vi "11.vi"() -> ()   [LabVIEW 2023]
uses:
  <vilib>/Utility/file.llb/Read Delimited Spreadsheet (string).vi
  <vilib>/Utility/file.llb/Write Delimited Spreadsheet (string).vi
panel:
  in  "stop":bool
  out "subarray 2":dbl[](array[numeric])
  out "x citit":dbl[](array[numeric])
  out "deleted portion":string[](array[string])
  out "array w/ subset deleted":string[][](array[string])
  out "XY Graph 2":cluster{dbl[], dbl[]}(graph)
  in  "desen":bool
  out "Y":dbl
  out "X":dbl
  out "subarray":string[](array[string])
  out "all rows":string[][](array[string])
  in  "citeste":bool
  in  "save":bool
  in  "b":dbl(slide) scale=0.0..10.0
  in  "a":dbl(slide) scale=0.0..10.0
  out "XY Graph":cluster{"X":dbl, "Y":dbl}[](graph)
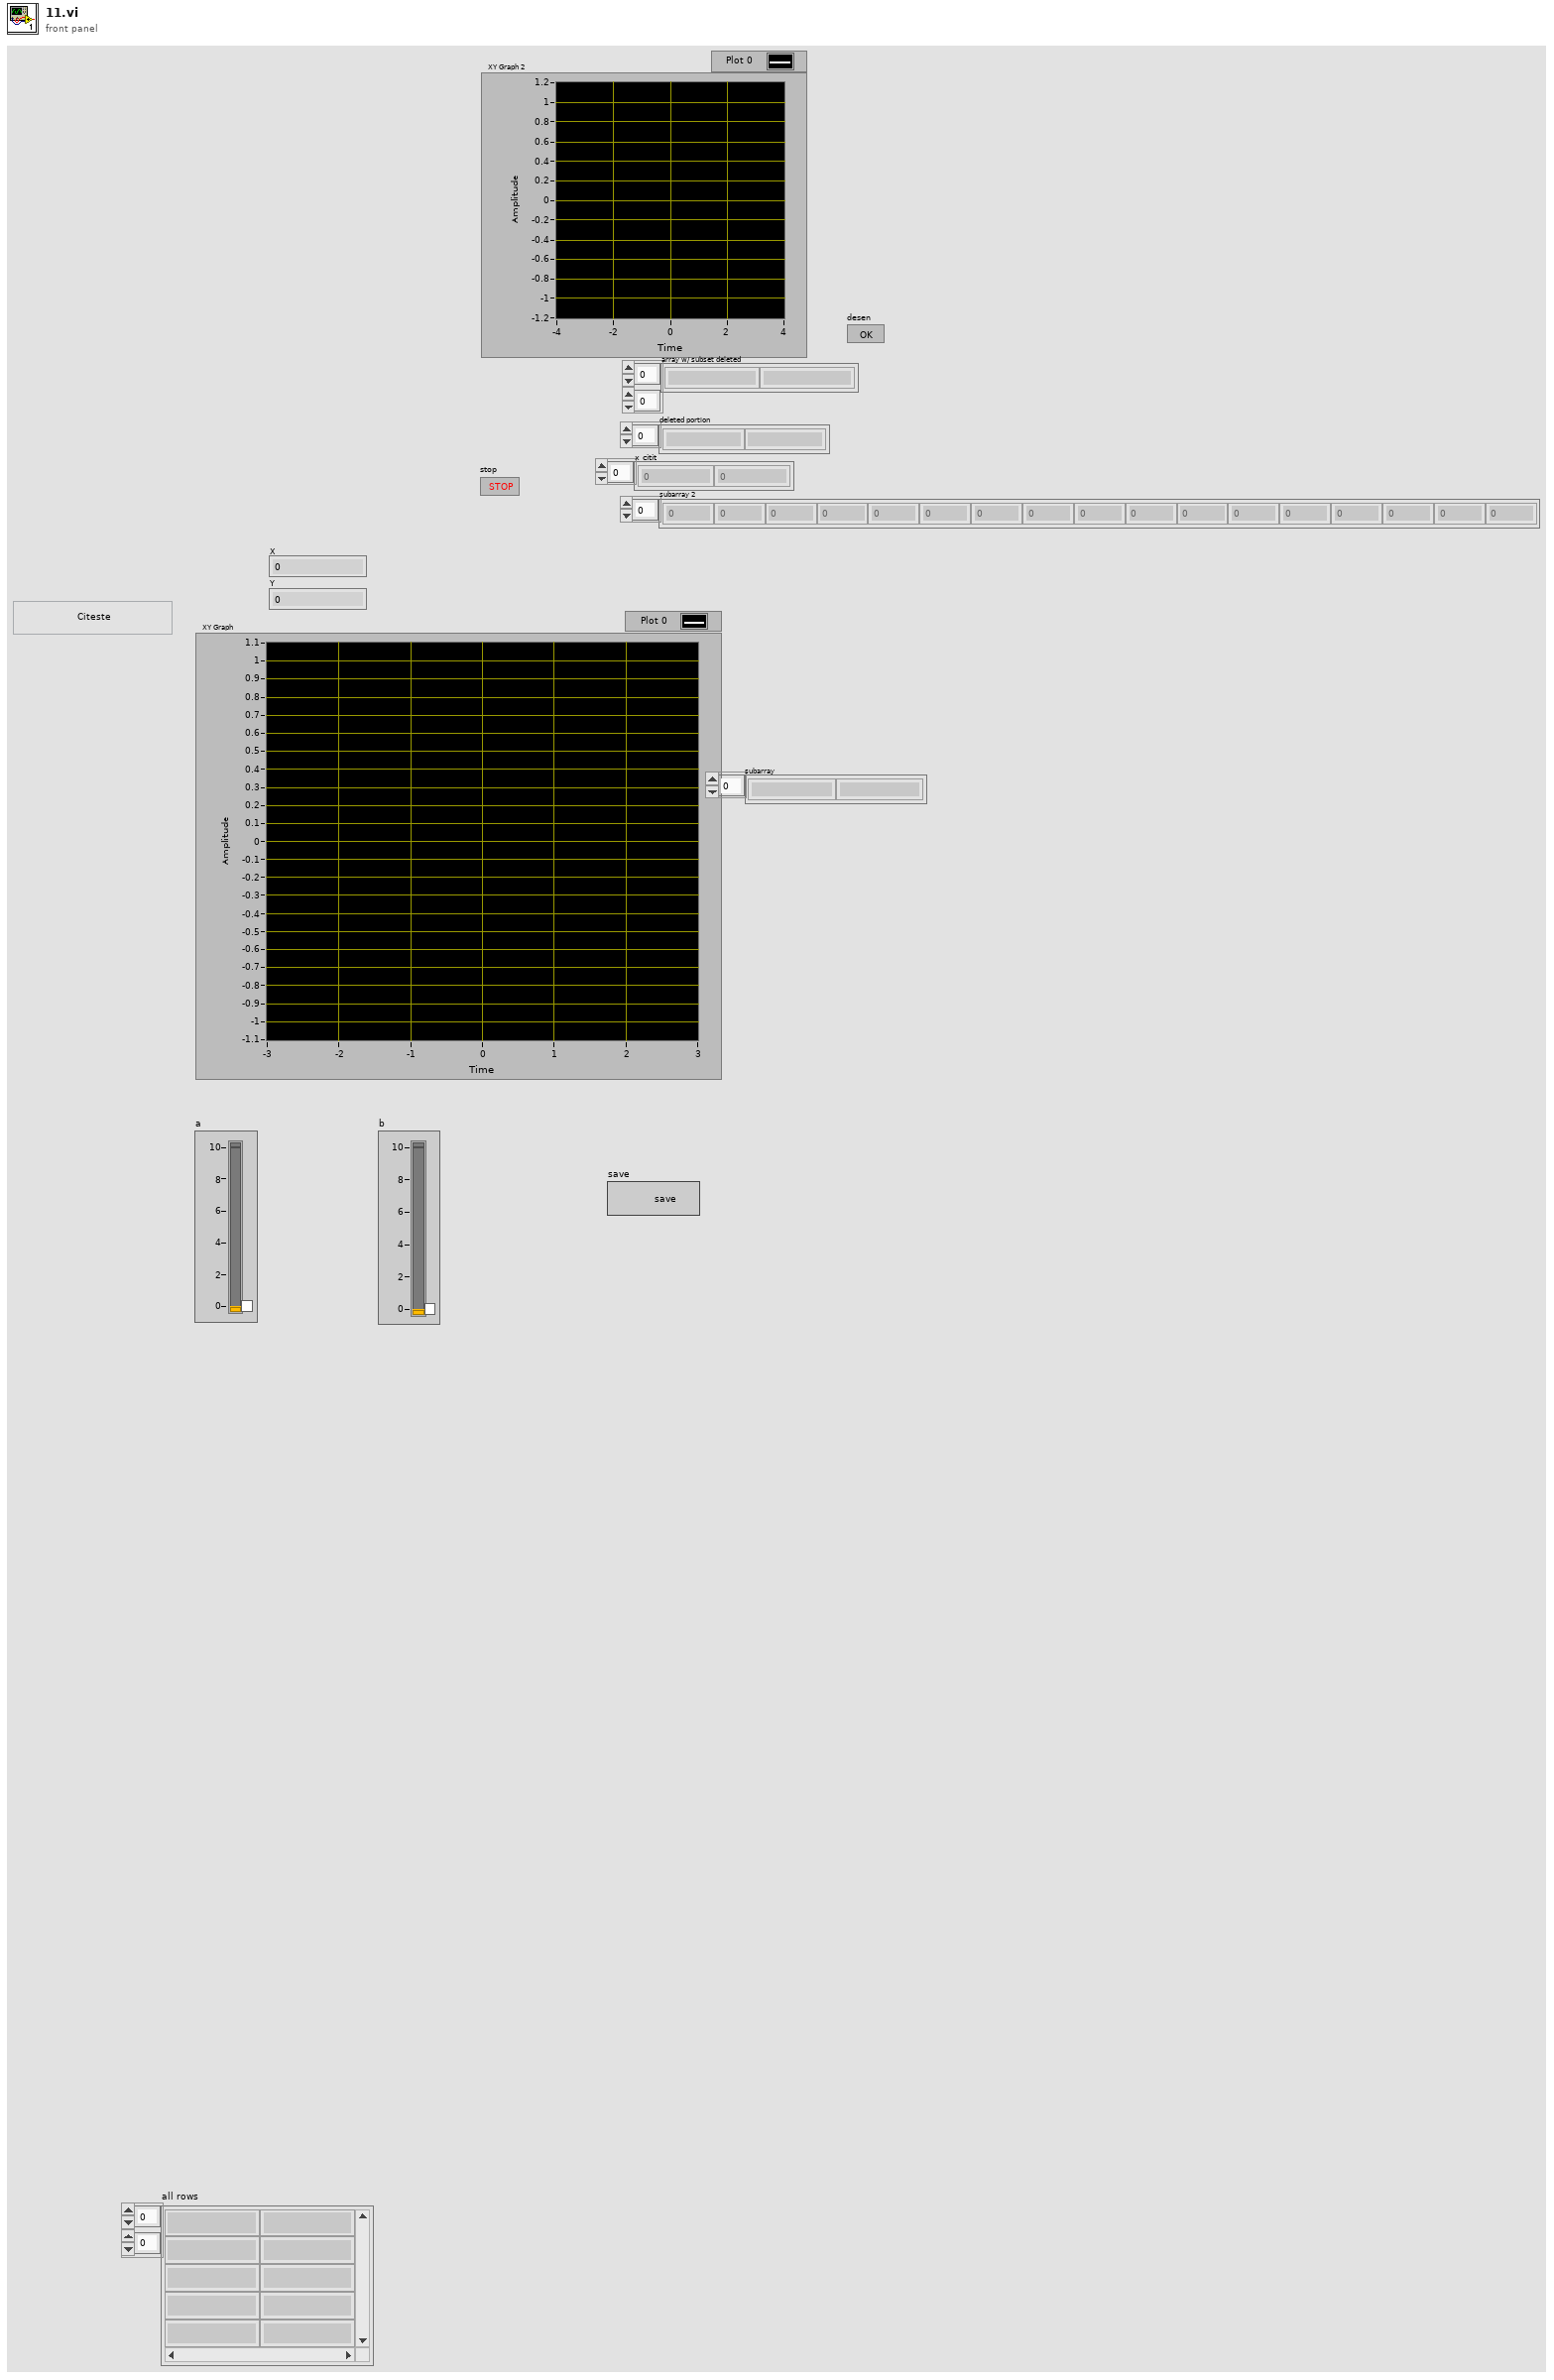
[diagram p1: front panel]
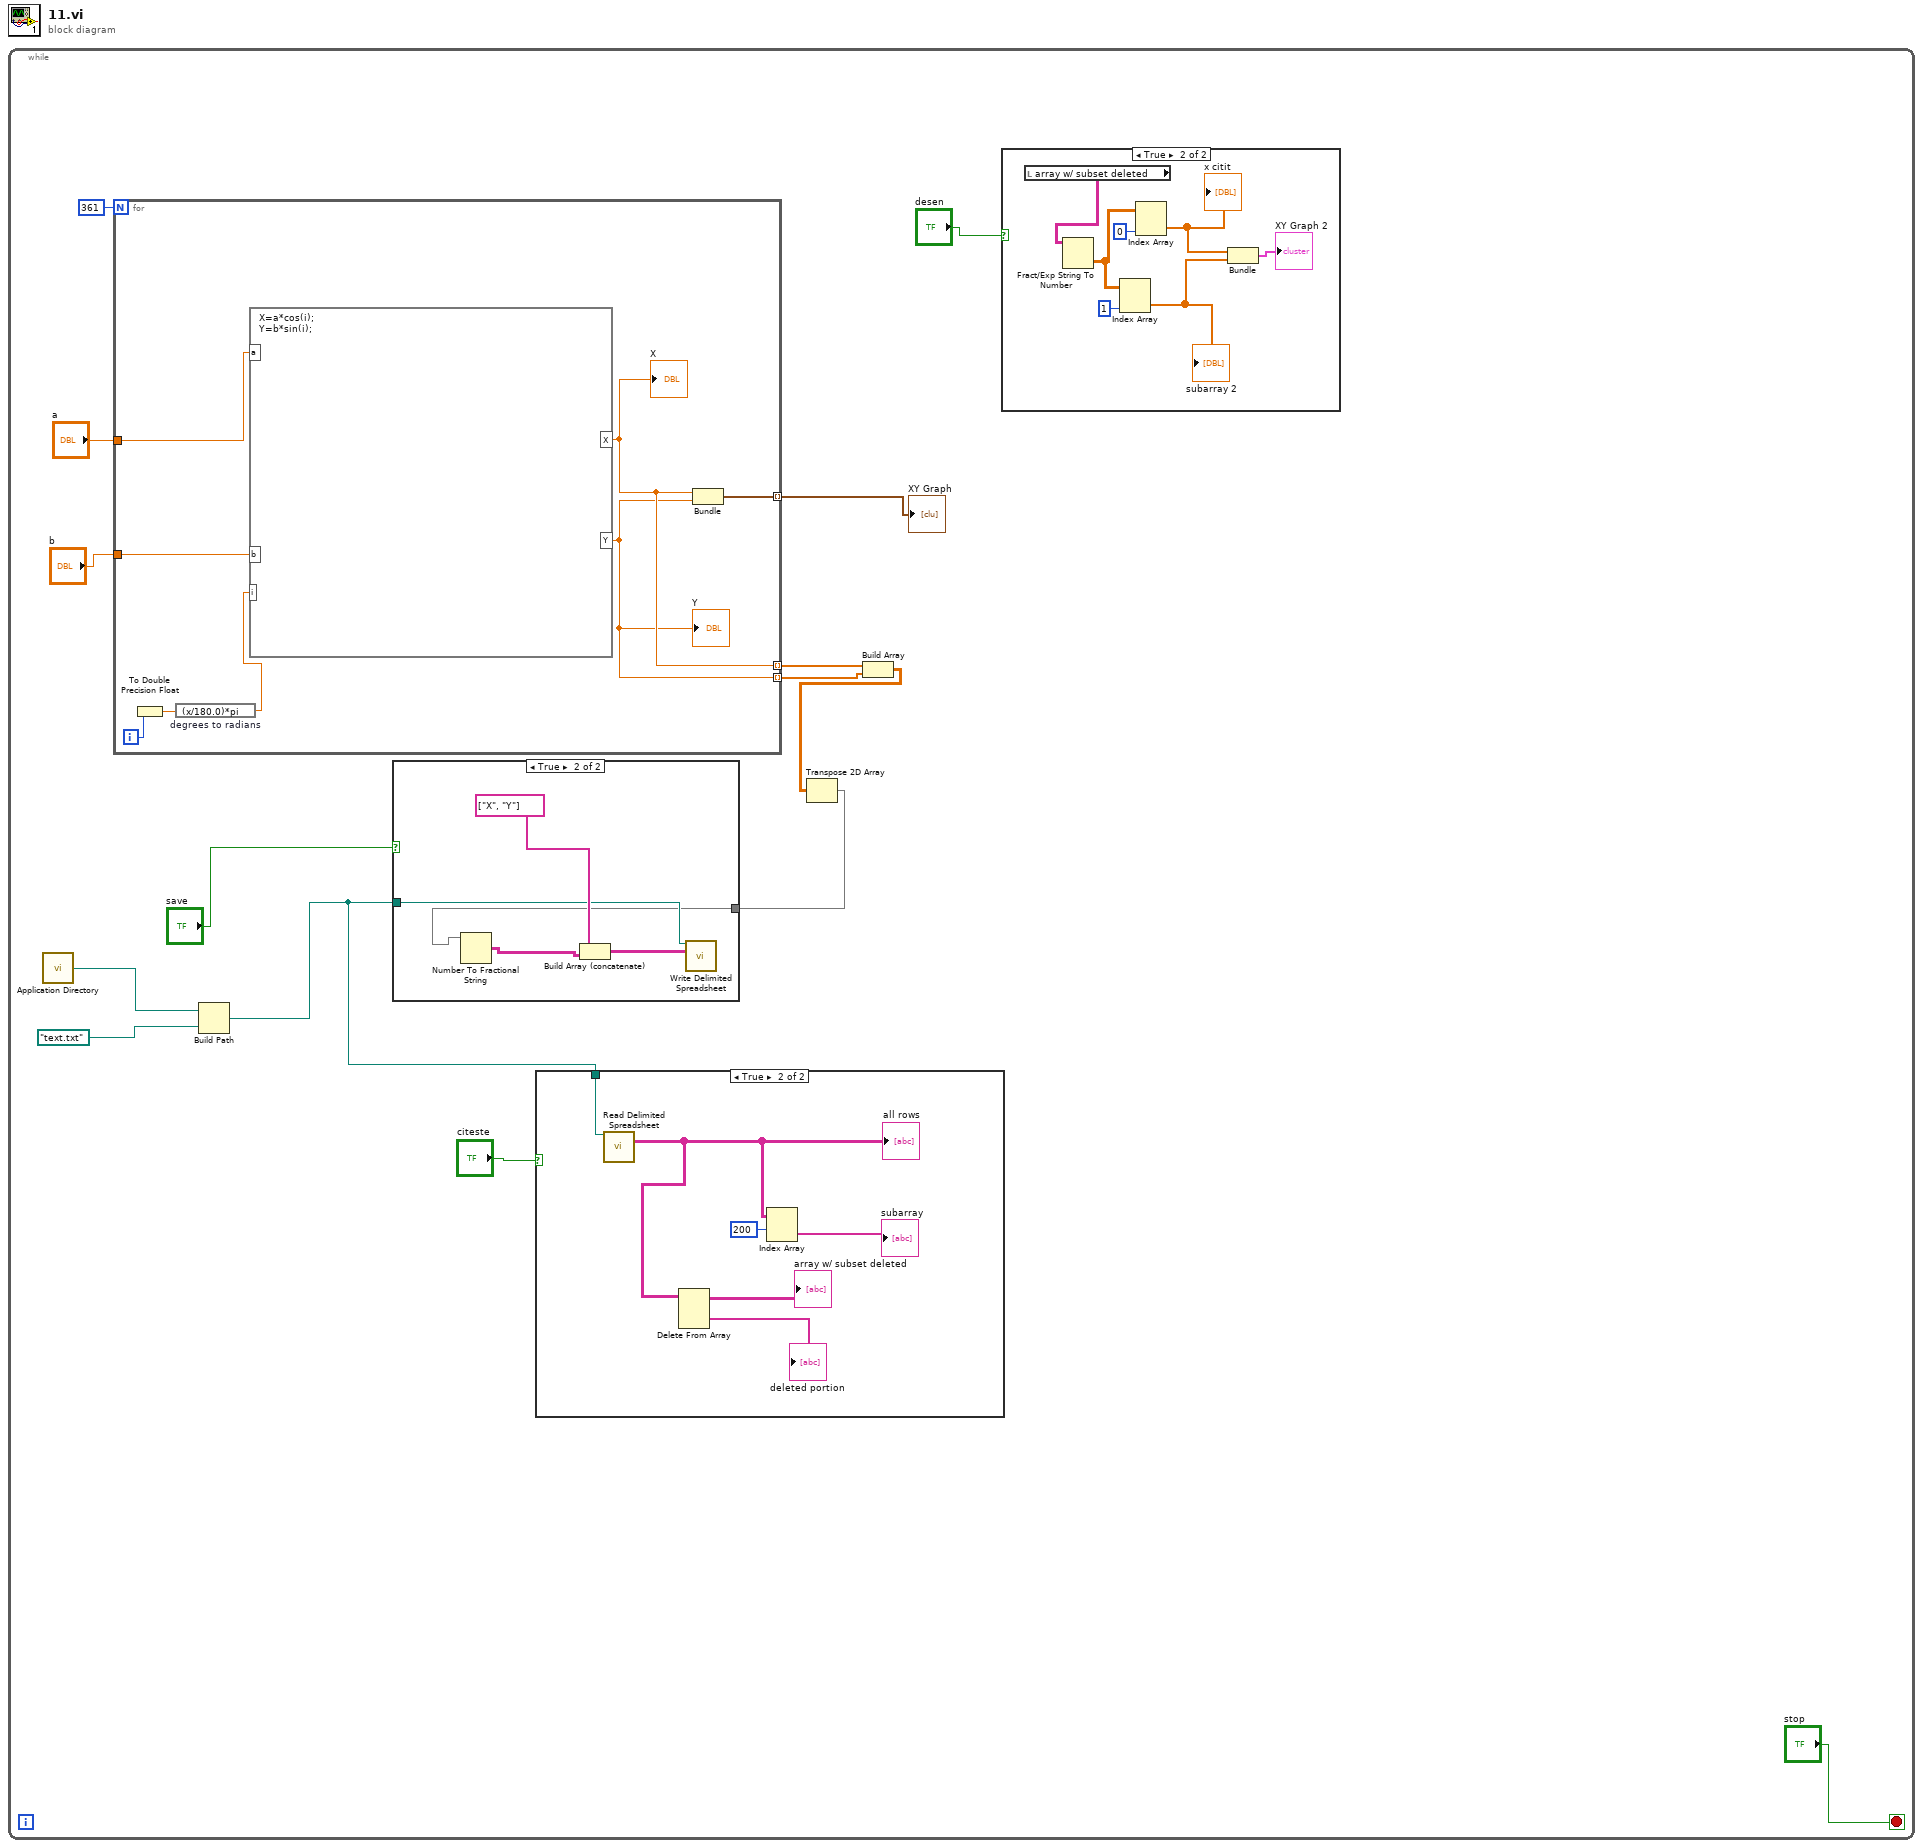
[diagram p0: block diagram]
diagram:
  n1 = while {
    stop <- "stop" stop-if-true
    n2 = call <vilib>:"Application Directory.vi"() -> ("Application Directory"=w9:path)
    n3 = for {
      N: 361 -> [_]
      tunnel: "a" -> [w41]
      tunnel: "b" -> [w40]
      tunnel: [w36] -> w13 mode=indexing
      tunnel: [w35] -> w8 mode=indexing
      tunnel: [w34] -> w7 mode=indexing
      i -> [w37]
      n4 = To Double Precision Float(number=w37) -> (double precision float=w38:dbl)
      n5 = expression code="(x/180.0)*pi" "degrees to radians"(w38) -> (w39:dbl)
      n6 = formula code="X=a*cos(i);\nY=b*sin(i);"("a"=w41, "b"=w40, "i"=w39) -> ("X"=w35:dbl, "Y"=w34:dbl)
      "X" <- w35
      "Y" <- w34
      n7 = Bundle("X"=w35, "Y"=w34) -> (w36:cluster{"X":dbl, "Y":dbl})  [unwired: 1 in]
    }
    "XY Graph" <- w13
    n8 = Build Path(base path=w9, name or relative path=path "text.txt") -> (appended path=w3:path)
    n9 = case shown="True" "citeste" {
      tunnel: w3 -> [_ w28]
      frame False {
      }
      frame True {
        n10 = call-poly <vilib>:"Read Delimited Spreadsheet.vi"("file path (dialog if empty)"=w28) -> ("all rows"=w25:string[][])  [unwired: 9 in, 5 out]
        "all rows" <- w25
        n11 = Delete From Array "Delete From Array"(array=w25) -> (deleted portion=→"deleted portion":string[], array with subset deleted=→"array w/ subset deleted":string[][])  [unwired: 3 in]
        n12 = Index Array "Index Array"(array=w25, index (row)=200) -> (element=→"subarray":string[])  [unwired: 1 in]
      }
    }
    n13 = Build Array(w8, w7) -> (w6:dbl[][])
    n14 = Transpose 2D Array(2D array=w6) -> (transposed array=w5:dbl[][])
    n15 = case shown="True" "save" {
      tunnel: w5 -> [_ w29]
      tunnel: w3 -> [_ w31]
      frame False {
      }
      frame True {
        n16 = Number To Fractional String(number=w29) -> (F-format string=w30:string[][])  [unwired: 3 in]
        n17 = Build Array (concatenate) "Build Array"(string[] ["X", "Y"] ("element"), w30) -> (w32:string[][])
        n18 = call-poly <vilib>:"Write Delimited Spreadsheet.vi"("file path (dialog if empty)"=w31, "2D data"=w32) -> ()  [unwired: 12 in, 2 out]
      }
    }
    n19 = case shown="True" "desen" {
      frame False {
      }
      frame True {
        n20 = local read "array w/ subset deleted"() -> (w22:string[][])
        n21 = Fract/Exp String To Number(string=w22) -> (number=w21:dbl[][])  [unwired: 3 in, 1 out]
        n22 = Index Array(array=w21, index (col)=1 ("disabled index (col)")) -> (element=w19:dbl[])  [unwired: 1 in]
        "subarray 2" <- w19
        n23 = Index Array(array=w21, index (col)=0 ("disabled index (col)")) -> (element=w20:dbl[])  [unwired: 1 in]
        "x citit" <- w20
        n24 = Bundle(w20, w19) -> (→"XY Graph 2":cluster{dbl[], dbl[]})  [unwired: 1 in]
      }
    }
  }
